vi "Toggle_case_VI.vi"() -> ()   [LabVIEW 2021]
doc: "This VI Toggles the characters entered.\nIf entered char is Upper case, then convereted to Lower case.\nIf entered char is Lower case, then convereted to Uower case."
panel:
  in  "Stop":bool
  in  "Input_String":string
  # "TOGGLE CASE GENERATOR"
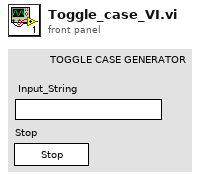
[diagram p1: front panel]
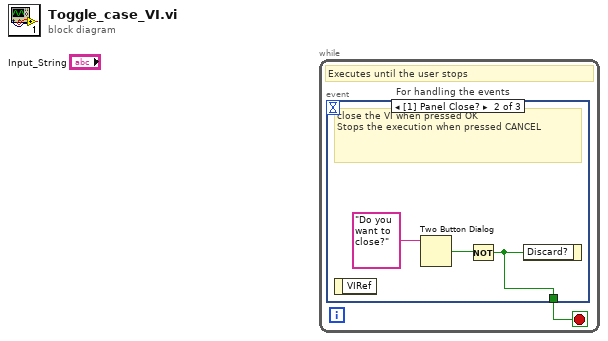
[diagram p0: block diagram]
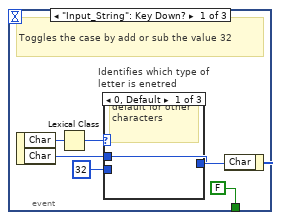
[diagram p2: hidden frame]
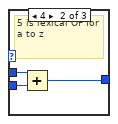
[diagram p3: hidden frame]
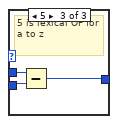
[diagram p4: hidden frame]
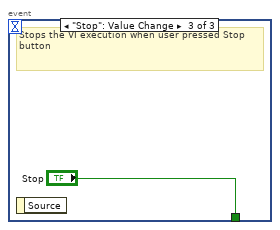
[diagram p5: hidden frame]
diagram:
  n1 = while {
    stop <- w1 stop-if-true
    # "Executes until the user stops"
    n2 = event "For handling the events" shown="[1] Panel Close?" {
      selector: _ -> [_ _ _]
      dyn-events: _ -> [_ _ _]
      timeout: _ -> [_ _ _]
      tunnel: [FALSE w15 "Stop"] -> w1
      event "Input_String": Key Down? {
        # "Toggles the case by add or sub the value 32"
        n3 = event-data() -> ("Char"=w7:i16, "Char"=w5:i16)  [unwired: 1 in]
        n4 = Lexical Class(1:w7) -> (0:w6:i16)
        n5 = case "Identifies which type of letter is enetred" shown="0, Default" w6 {
          tunnel: [w8 w11 w14] -> w4
          tunnel: w5 -> [w8 w10 w13]
          tunnel: i16 32 -> [_ w9 w12]
          frame 0, Default {
            # "default for other characters"
          }
          frame 4 {
            # "5 is lexical OP for a to z"
            n6 = Add(x=w10, y=w9) -> (x+y=w11:i16)
          }
          frame 5 {
            # "5 is lexical OP for a to z"
            n7 = Subtract(x=w13, y=w12) -> (x-y=w14:i16)
          }
        }
        n8 = event-data("Char"=w4) -> ()  [unwired: 1 in, 1 out]
      }
      event Panel Close? {
        # "close the VI when pressed OK\nStops the execution when pressed CANCEL"
        n9 = event-data() -> ()  [unwired: 1 in, 1 out]
        n10 = Two Button Dialog(message="Do you want to close?") -> (T button?=w16:bool)  [unwired: 2 in]
        n11 = Not(x=w16) -> (.not. x?=w15:bool)
        n12 = event-data("Discard?"=w15) -> ()  [unwired: 1 in, 1 out]
      }
      event "Stop": Value Change {
        # "Stops the VI execution when user pressed Stop button"
        n13 = event-data() -> ()  [unwired: 1 in, 1 out]
      }
    }
  }
